vi "prepareDAPCParameters.vi"(8 "error in (no error)":errorcluster, 11 "TestDataLog in":refnum<class "TestDataLog.lvclass">) -> (0 "error out":errorcluster, 2 "DualActingPneumaticCylinderParameters":string, 3 "TestDataLog out":refnum<class "TestDataLog.lvclass">)   [LabVIEW 2013, in "TestDataLog.lvclass"]
uses:
  TestDataLog.lvclass
  TestDataLog.lvclass/TestDataLog.ctl
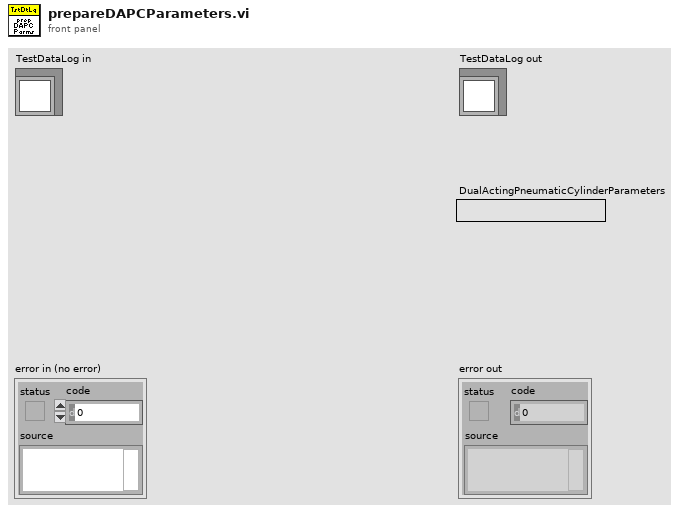
[diagram p1: front panel]
types:
  T1 = typedef "FAMTTypedefs.lvlib/DualActingPneumaticCylinder.ctl" = cluster{"Pressure Transducer Compensator":T2, "Flow Control Valve Compensator":T5}
  T2 = typedef "PressureTransducerCompensator.ctl" = cluster{"PID Gains":T3, "Pressure Transducer Output Range":T4, "Vcoil":dbl[unit]}
  T3 = typedef "PIDGains.ctl" = cluster{"Proportional Gain (Kc)":dbl, "Integral Time (Ti, min)":dbl, "Derivative Time (Td, min)":dbl}
  T4 = typedef "PressureTransducerOutputRange.ctl" = cluster{"High":dbl[unit], "Low":dbl[unit]}
  T5 = typedef "FlowControlValveCompensator.ctl" = cluster{"PID Gains":T3, "Flow Control Valve Output Range":T6}
  T6 = typedef "FlowControlValveOutputRange.ctl" = cluster{"High":dbl[unit], "Low":dbl[unit]}
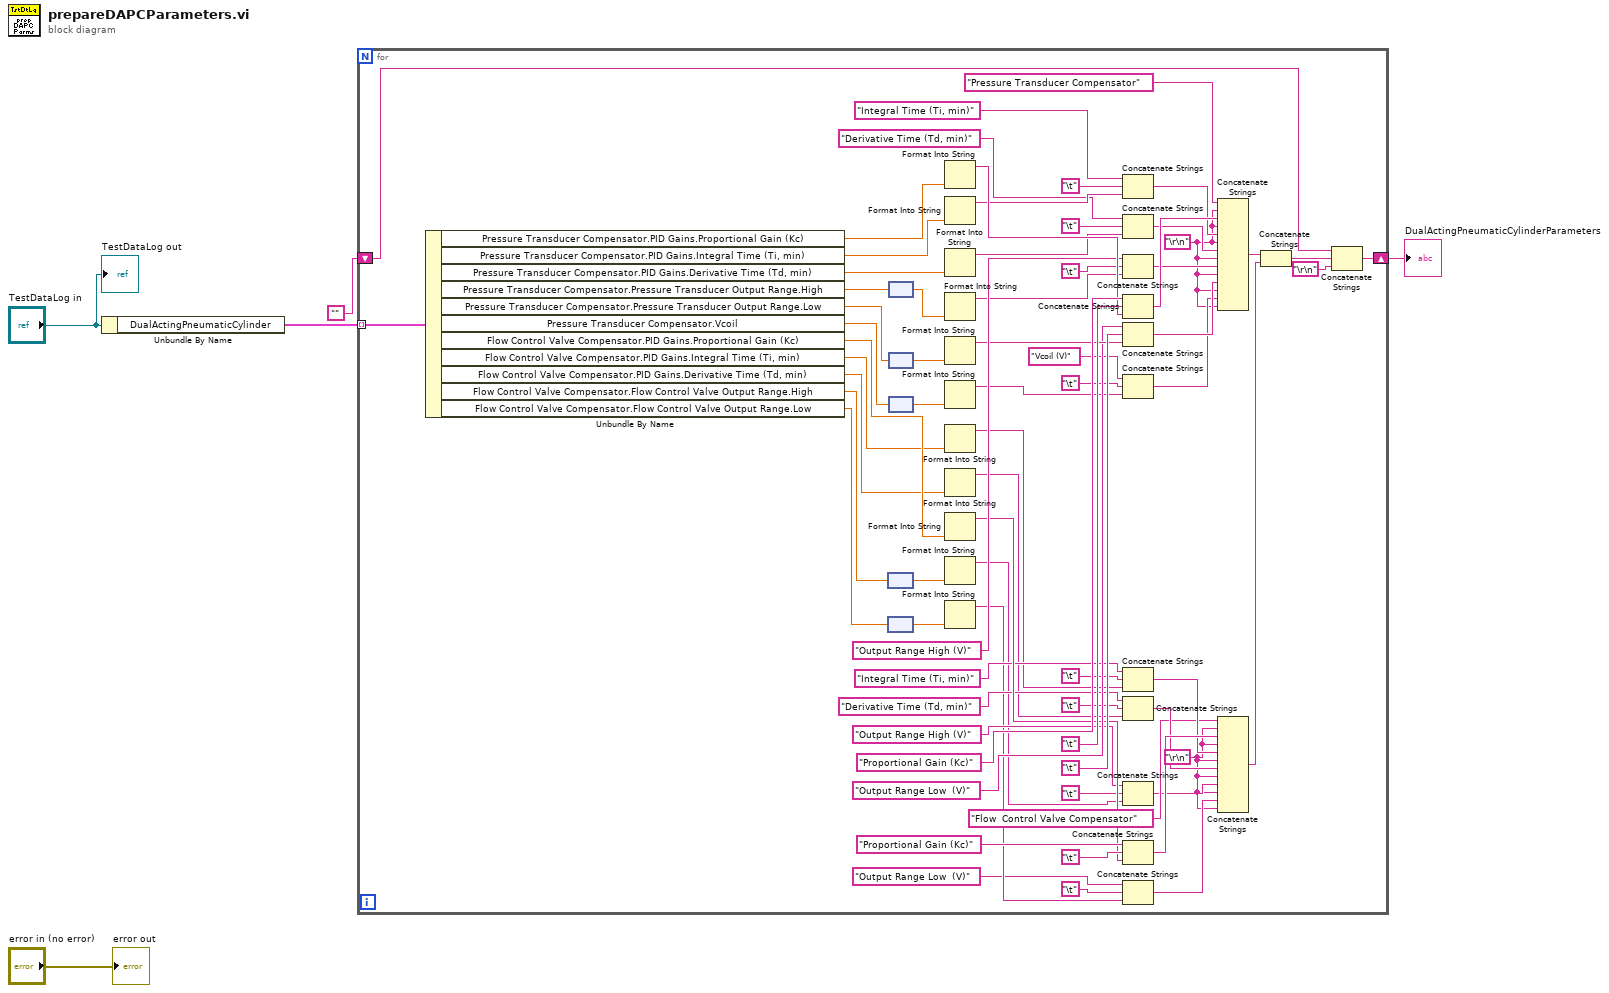
[diagram p0: block diagram]
diagram:
  n1 = Unbundle By Name("TestDataLog in") -> ("DualActingPneumaticCylinder"=w4:T1[])
  n2 = for {
    tunnel: w4 -> [w68] mode=indexing
    shift-right: [w7] -> w1
    shift-left: "" -> [w9]
    w25 = "\r\n"
    w12 = "\r\n"
    n3 = Unbundle By Name(w68) -> ("Pressure Transducer Compensator.PID Gains.Proportional Gain (Kc)"=w65:dbl, "Pressure Transducer Compensator.PID Gains.Integral Time (Ti, min)"=w63:dbl, "Pressure Transducer Compensator.PID Gains.Derivative Time (Td, min)"=w64:dbl, "Pressure Transducer Compensator.Pressure Transducer Output Range.High"=w56:dbl[unit], "Pressure Transducer Compensator.Pressure Transducer Output Range.Low"=w51:dbl[unit], "Pressure Transducer Compensator.Vcoil"=w17:dbl[unit], "Flow Control Valve Compensator.PID Gains.Proportional Gain (Kc)"=w23:dbl, "Flow Control Valve Compensator.PID Gains.Integral Time (Ti, min)"=w22:dbl, "Flow Control Valve Compensator.PID Gains.Derivative Time (Td, min)"=w21:dbl, "Flow Control Valve Compensator.Flow Control Valve Output Range.High"=w20:dbl[unit], "Flow Control Valve Compensator.Flow Control Valve Output Range.Low"=w19:dbl[unit])
    n4 = node(w20) -> (w31:dbl)
    n5 = node(w19) -> (w30:dbl)
    n6 = node(w56) -> (w55:dbl)
    n7 = node(w51) -> (w54:dbl)
    n8 = node(w17) -> (w16:dbl)
    n9 = Format Into String(w65) -> (resulting string=w73:string)  [unwired: 3 in, 1 out]
    n10 = Format Into String(w63) -> (resulting string=w71:string)  [unwired: 3 in, 1 out]
    n11 = Format Into String(w64) -> (resulting string=w69:string)  [unwired: 3 in, 1 out]
    n12 = Format Into String(w55) -> (resulting string=w53:string)  [unwired: 3 in, 1 out]
    n13 = Format Into String(w54) -> (resulting string=w52:string)  [unwired: 3 in, 1 out]
    n14 = Format Into String(w16) -> (resulting string=w15:string)  [unwired: 3 in, 1 out]
    n15 = Format Into String(w22) -> (resulting string=w42:string)  [unwired: 3 in, 1 out]
    n16 = Format Into String(w21) -> (resulting string=w40:string)  [unwired: 3 in, 1 out]
    n17 = Format Into String(w23) -> (resulting string=w44:string)  [unwired: 3 in, 1 out]
    n18 = Format Into String(w31) -> (resulting string=w29:string)  [unwired: 3 in, 1 out]
    n19 = Format Into String(w30) -> (resulting string=w28:string)  [unwired: 3 in, 1 out]
    n20 = Concatenate Strings("Integral Time (Ti, min)" ("element"), "\t", w71) -> (w66:string)
    n21 = Concatenate Strings("Derivative Time (Td, min)" ("element"), "\t", w69) -> (w62:string)
    n22 = Concatenate Strings("Output Range High (V)" ("element"), "\t", w53) -> (w50:string)
    n23 = Concatenate Strings("Proportional Gain (Kc)" ("element"), "\t", w73) -> (w67:string)
    n24 = Concatenate Strings("Output Range Low  (V)" ("element"), "\t", w52) -> (w49:string)
    n25 = Concatenate Strings("Vcoil (V)" ("string"), "\t", w15) -> (w13:string)
    n26 = Concatenate Strings("Integral Time (Ti, min)" ("element"), "\t", w42) -> (w38:string)
    n27 = Concatenate Strings("Derivative Time (Td, min)" ("element"), "\t", w40) -> (w37:string)
    n28 = Concatenate Strings("Output Range High (V)" ("element"), "\t", w29) -> (w27:string)
    n29 = Concatenate Strings("Proportional Gain (Kc)" ("element"), "\t", w44) -> (w39:string)
    n30 = Concatenate Strings("Output Range Low  (V)" ("element"), "\t", w28) -> (w26:string)
    n31 = Concatenate Strings("Pressure Transducer Compensator" ("string"), w12, w67, w12, w66, w12, w62, w12, w50, w12, w49, w12, w13, w12) -> (w11:string)
    n32 = Concatenate Strings("Flow  Control Valve Compensator" ("string"), w25, w39, w25, w38, w25, w37, w25, w27, w25, w26, w25) -> (w10:string)
    n33 = Concatenate Strings(w11, w10) -> (w8:string)
    n34 = Concatenate Strings(w9, w8, "\r\n") -> (w7:string)
  }
  "DualActingPneumaticCylinderParameters" <- w1
  "error out" <- "error in (no error)"
  "TestDataLog out" <- "TestDataLog in"
